vi "clearSoundDevice.vi"(0 "Sound Device OUT":T3 {"task ID" format="%.0x"}) -> ()   [LabVIEW 2010]
uses:
  <vilib>/sound2/lvsound2.llb/Sound Output Task ID.ctl
  <vilib>/sound2/lvsound2.llb/Sound Data Format.ctl
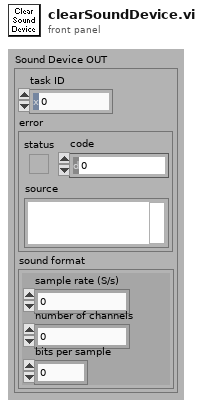
[diagram p1: front panel]
types:
  T1 = typedef "Sound Output Task ID.ctl" = u32
  T2 = typedef "Sound Data Format.ctl" = cluster{"sample rate (S/s)":dbl, "number of channels":i32, "bits per sample":i32}
  T3 = cluster{"task ID":T1, "error":errorcluster, "sound format":T2}
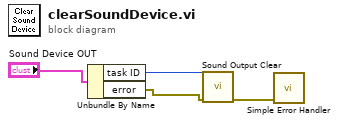
[diagram p0: block diagram]
diagram:
  n1 = Unbundle By Name("Sound Device OUT") -> ("task ID"=w1:T1, "error"=w2:errorcluster)
  n2 = call <vilib>:"Sound Output Clear.vi"("error in (no error)"=w2, "task ID"=w1) -> ("error out"=w4:errorcluster)  [unwired: 9 in]
  n3 = call <vilib>:"Simple Error Handler.vi"("error in (no error)"=w4) -> ()  [unwired: 4 in, 5 out]
